vi "Count Up.vi"(7 "Reset?":bool, 11 "goal":u32) -> (3 "Count Met":bool, 5 "count":u32)   [LabVIEW 2012]
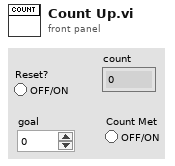
[diagram p1: front panel]
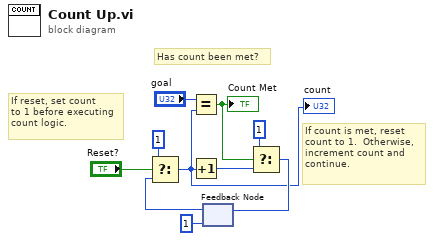
[diagram p0: block diagram]
diagram:
  # "If reset, set count \nto 1 before executing\ncount logic."
  # "If count is met, reset \ncount to 1.  Otherwise,\nincrement count and \ncontinue."
  # "Has count been met?"
  n1 = feedback #1(u32 1 ("f")) -> (w5:u32)
  n2 = Select(t=u32 1, s="Reset?", f=w5) -> (s? t:f=w2:u32)
  "count" <- w2
  n3 = Equal?(x="goal", y=w2) -> (x = y?=w1:bool)
  "Count Met" <- w1
  n4 = Increment(x=w2) -> (x+1=w8:u32)
  n5 = Select(t=u32 1 ("f"), s=w1, f=w8) -> (s? t:f=w10:u32)
  n6 = feedback-in #1(w10) -> ()
